vi "Query Blender Overrun Status.vi"(8 "error in (no error)":errorcluster, 10 "Blender (1)":u32 min=1 max=2 step=1, 11 "VISA resource name":refnum<visa-resource-name>) -> (0 "error out":errorcluster, 2 "Overrun Status":i32, 3 "VISA resource name out":refnum<visa-resource-name>)   [LabVIEW 2009, in "Keithley DMM7510.lvlib"]
doc: "This VI returns the event detector overrun status."
uses:
  Keithley DMM7510.lvlib
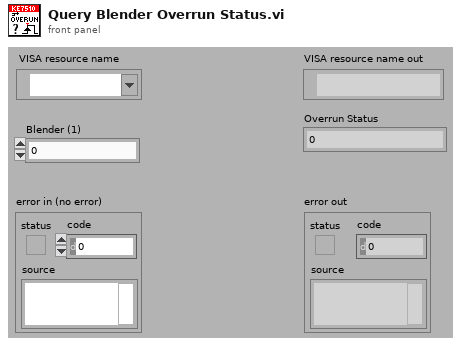
[diagram p1: front panel]
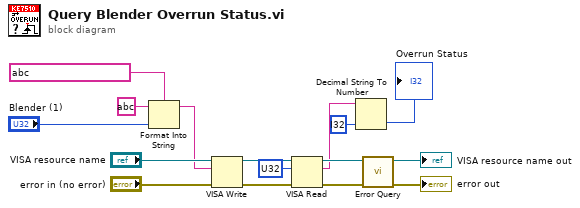
[diagram p0: block diagram]
diagram:
  n1 = Format Into String(format string=string ?, initial string=string ?, "Blender (1)") -> (resulting string=w5:string)  [unwired: 1 in, 1 out]
  n2 = VISA Write(VISA resource name="VISA resource name", write buffer=w5, error in (no error)="error in (no error)") -> (VISA resource name out=w10:refnum<visa-resource-name>, error out=w12:errorcluster)  [unwired: 1 out]
  n3 = VISA Read(VISA resource name=w10, byte count=u32 ?, error in (no error)=w12) -> (VISA resource name out=w9:refnum<visa-resource-name>, read buffer=w4:string, error out=w11:errorcluster)  [unwired: 1 out]
  n4 = Decimal String To Number(string=w4, default (0L)=i32 ? ("default (0 I32)")) -> (number=→"Overrun Status":i32)  [unwired: 1 in, 1 out]
  n5 = call "Error Query.vi"("error in (no error)"=w11, "VISA resource name"=w9) -> ("error out"=→"error out":errorcluster, "VISA resource name out"=→"VISA resource name out":refnum<visa-resource-name>)  [unwired: 8 out]
